vi "PH_PowerUnit_BaseClass.PC_TrendMssgs.vi"(0 "i ref in":refnum<vi>, 2 "Instance":string, 3 "Status":T1 items=["no info", "off/false/out", "on/true/in", "Failure", "Alarm", "Status 1", "Status 2", "Status 3"], 4 "not linked?":bool, 5 "error in (no error)":errorcluster) -> (14 "i ref out":refnum<vi>, 19 "error out":errorcluster)   [LabVIEW 2014, in "PH_PowerUnit_BaseClass.lvlib"]
doc: "This VI writes the incoming information to own attributes."
uses:
  PH_PowerUnit_BaseClass.lvlib
  PH_StatusHandler/PH_StatusHandler.Status.ctl
  PH_Common/PH_Common.lvlib
  PH_StatusHandler/PH_StatusHandler.lvlib
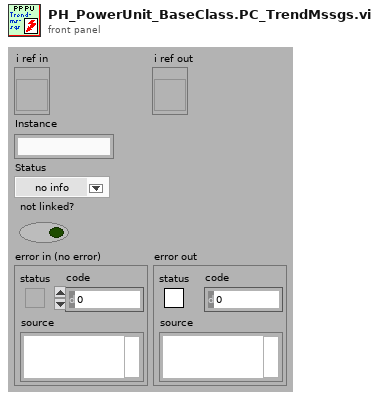
[diagram p1: front panel]
types:
  T1 = typedef "PH_StatusHandler.lvlib/PH_StatusHandler.Status.ctl" = i16
  T2 = typedef "PH_PowerUnit_BaseClass.lvlib/PH_PowerUnit_BaseClass.i attribute.ctl" = cluster{"Constructor finished":bool, "PU":cluster{"In use":bool, "Service ID in use":i32, "GUI Ref":refnum<vi>}, "Enabling":cluster{"State":T3, "GUI Ref":refnum<vi>}, "Timing":cluster{"Last Shot":dbl, "Time between Shots [Sec]":dbl, "Waiting Time over?":bool, "Service ID Waiting Time":i32, "GUI Ref":refnum<vi>, "Instance":cluster{"Status":T1, "linked?":bool, "GUI Ref":refnum<vi>}}, "Sequencer":cluster{"SM State":string, "GUI Ref":refnum<vi>, "linked":bool}, "Subscribed Trendmssgs":cluster{"Tagname":string, "Status":T1, "linked?":bool, "Shot Condition":T1, "GUI Ref":refnum<vi>}[], "PP PU":T4, "Default Voltage (V)":dbl, "GUI Refs":T5, "PSDB data":cluster{"Shot Voltage [V]":dbl, "State TO SM":T6, "Write 2 early":bool}, "State TO SM":T6}
  T3 = typedef "PH_SystemInformation.lvlib/PH_SystemInformationEnabling State.ctl" = i32
  T4 = typedef "PH_PP_Common.lvlib/PH_PP_Common.PUs.ctl" = enum16{"no Info", "PA-19mm-1", "PA-19mm-2", "PA-45mm-PILC", "PA-45mm-MAIN", "MA-PU-1", "MA-PU-2", "MA-PU-3", "MA-PU-4", "MA-PU-5", "MA-PU-6", "MA-FR", "MA-PILC", "PA-45mm-DP"}
  T5 = typedef "PH_PowerUnit_BaseClass.lvlib/PH_PowerUnit_BaseClass.GUI Refs.ctl" = cluster{"Delete Inst":refnum<vi>, "State TO SM":refnum<vi>, "State SM":refnum<vi>, "Fire":refnum<vi>}
  T6 = typedef "PH_PowerUnit_BaseClass.lvlib/PH_PowerUnit_BaseClass.SM States.ctl" = enum16{".", "Stand by", "Switch PU on", "Configure", "Set Default Voltage", "Set STANDBY", "Set READY", "Wait for Shot Cmd", "Open Dump Rods", "Open Ross Relais", "Close Ross Relais", "Switch PSU on", "Switch PSU off", "Charge", "Switch GD Channel on", "Close Dump Rods", "Rods-TO", "RR-TO", "PSU-TO", "Trigger-TO"}
  T7 = cluster{"Tagname":string, "Status":T1, "linked?":bool, "Shot Condition":T1, "GUI Ref":refnum<vi>}[]
  T8 = cluster{"Tagname":string, "Status":T1, "linked?":bool, "Shot Condition":T1, "GUI Ref":refnum<vi>}
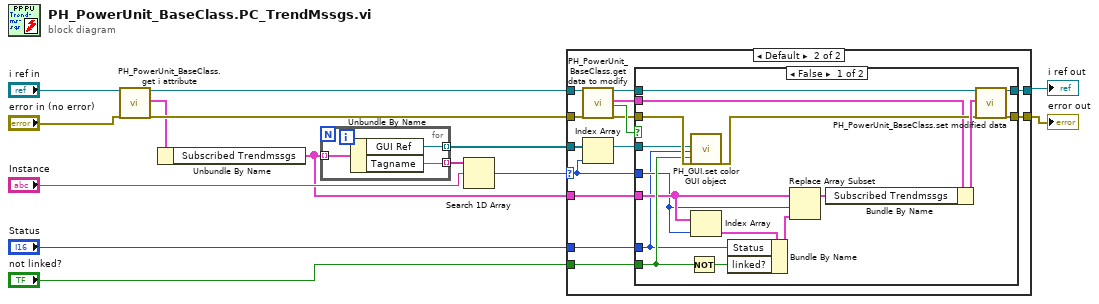
[diagram p0: block diagram]
diagram:
  n1 = call "PH_PowerUnit_BaseClass.get i attribute.vi"("i ref in"="i ref in", "error in (no error)"="error in (no error)") -> ("i ref out"=w7:refnum<vi>, "i attribute"=w6:T2, "error out"=w9:errorcluster)  [unwired: 15 in]
  n2 = Unbundle By Name(w6) -> ("Subscribed Trendmssgs"=w1:T7)
  n3 = for {
    tunnel: w1 -> [w17] mode=indexing
    tunnel: [w16] -> w5 mode=indexing
    tunnel: [w15] -> w2 mode=indexing
    n4 = Unbundle By Name(w17) -> ("GUI Ref"=w15:refnum<vi>, "Tagname"=w16:string)
  }
  n5 = Search 1D Array(1D array=w5, element="Instance") -> (index of element=w3:i32)  [unwired: 1 in]
  n6 = case shown="Default" w3 {
    selector: w3 -> [_ w20]
    tunnel: [w18 w32] -> w13
    tunnel: [w19 w30] -> w12
    tunnel: "Status" -> [_ w27]
    tunnel: "not linked?" -> [_ w26]
    tunnel: w9 -> [w18 w25]
    tunnel: w7 -> [w19 w24]
    tunnel: w2 -> [_ w23]
    tunnel: w1 -> [_ w21]
    frame -1 {
    }
    frame Default {
      n7 = call "PH_PowerUnit_BaseClass.get data to modify.vi"("i ref in"=w24, "error in (no error)"=w25) -> ("i ref out"=w29:refnum<vi>, "i attribute"=w28:T2, "timed out"=w33:bool, "error out"=w31:errorcluster)  [unwired: 14 in]
      n8 = Index Array(array=w23, index=w20) -> (element=w22:refnum<vi>)
      n9 = case shown="False" w33 {
        tunnel: w29 -> [w49 w51]
        tunnel: [w46 w51] -> w30
        tunnel: w31 -> [w45 w50]
        tunnel: [w47 w50] -> w32
        tunnel: w28 -> [w41 _]
        tunnel: w27 -> [w35 _]
        tunnel: w26 -> [w43 _]
        tunnel: w22 -> [w42 _]
        tunnel: w21 -> [w39 _]
        tunnel: w20 -> [w38 _]
        frame False {
          n10 = Not(x=w43) -> (.not. x?=w34:bool)
          n11 = call "PH_GUI.set color GUI object.vi"("GUI object Ref"=w42, "State"=w35, "Blinking? (false)"=w43, "error in (no error)"=w45) -> ("error out"=w44:errorcluster)  [unwired: 15 in]
          n12 = Index Array(array=w39, index=w38) -> (element=w37:T8)
          n13 = Bundle By Name(cluster=w37, "Status"=w35, "linked?"=w34) -> (w36:T8)
          n14 = Replace Array Subset(array=w39, new element=w36, index=w38) -> (w40:T7)
          n15 = Bundle By Name(cluster=w41, "Subscribed Trendmssgs"=w40) -> (w48:T2)
          n16 = call "PH_PowerUnit_BaseClass.set modified data.vi"("i ref in"=w49, "i attribute"=w48, "error in (no error)"=w44) -> ("i ref out"=w46:refnum<vi>, "error out"=w47:errorcluster)  [unwired: 15 in]
        }
        frame True {
        }
      }
    }
  }
  "error out" <- w13
  "i ref out" <- w12
